vi "MotionProfileHandler.vi"(7 "Goal":dbl, 8 "MaxAccel":dbl=2.0 format="%#_13g", 9 "MaxVel":dbl=1.2 format="%#_13g", 10 "X":T1, 11 "Time":dbl) -> (3 "Goal":T1)   [LabVIEW 2017]
uses:
  <vilib>/Analysis/Matrix/Datatypes/RealMatrix.ctl
  <vilib>/Analysis/Matrix/NI_Matrix.lvlib
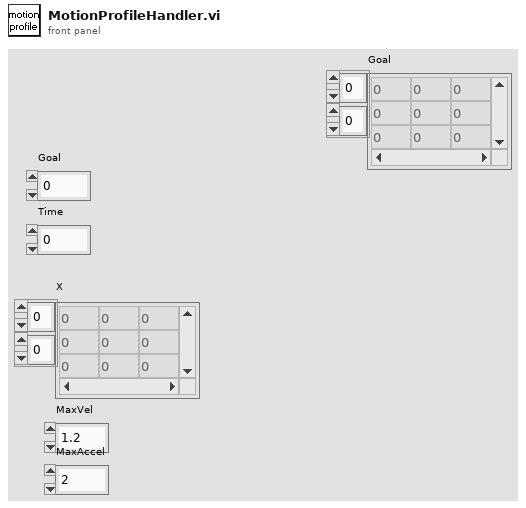
[diagram p1: front panel]
types:
  T1 = typedef "NI_Matrix.lvlib/RealMatrix.ctl" = dbl[][]
  T2 = cluster{"TargetPos":dbl, "InitalPos":dbl, "FinalVel":dbl, "IntitialVel":dbl, "MaxVel":dbl, "MaxAccel":dbl}
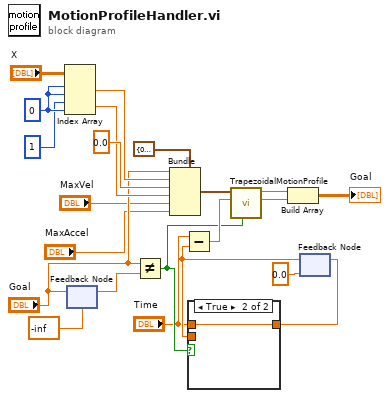
[diagram p0: block diagram]
diagram:
  w19 = 0 ("index (row)")
  n1 = Index Array(array="X", index (row) #1=w19, index (col) #1=w19, index (row) #2=1 ("index (row)"), index (col) #2=w19) -> (element #1=w16:dbl, element #2=w15:dbl)
  n2 = feedback #1(-inf ("Goal")) -> (w14:dbl)
  n3 = feedback-in #1("Goal") -> ()
  n4 = Not Equal?(x="Goal", y=w14) -> (x != y?=w3:bool)
  n5 = Bundle(cluster=T2 {"TargetPos"=0.0, "InitalPos"=0.0, "FinalVel"=0.0, "IntitialVel"=0.0, "MaxVel"=0.0, "MaxAccel"=0.0} ("Config"), "TargetPos"="Goal", "InitalPos"=w16, "FinalVel"=0.0, "IntitialVel"=w15, "MaxVel"="MaxVel", "MaxAccel"="MaxAccel") -> (w4:T2)
  n6 = feedback #2(0.0 ("Time")) -> (w21:dbl)
  n7 = Subtract(x="Time", y=w21) -> (x-y=w9:dbl)
  n8 = case shown="True" w3 {
    tunnel: [w23 w24] -> w22
    tunnel: w21 -> [w23 _]
    tunnel: "Time" -> [_ w24]
    frame False {
    }
    frame True {
    }
  }
  n9 = call "TrapezoidalMotionProfile.vi"("Initialize"=w3, "Time"=w9, "Config"=w4) -> ("Velocity"=w11:dbl, "Distance"=w12:dbl)  [unwired: 6 in, 1 out]
  n10 = Build Array(w12, w11) -> (→"Goal":T1)
  n11 = feedback-in #2(w22) -> ()
